vi "Periodic Tasks-Teleop Swerve.vi"(8 "error in":errorcluster) -> ()   [LabVIEW 2015]
doc: "This VI runs in parallel to other tasks. It can contain as many user-defined periodic loops as you need. These can carry out PID or other sorts of timed response."
uses:
  Robot Global Data.vi
  <vilib>/Rock Robotics/Network Tables/NT Read Number.vi
panel:
  out "Avg Absolute Distance":dbl
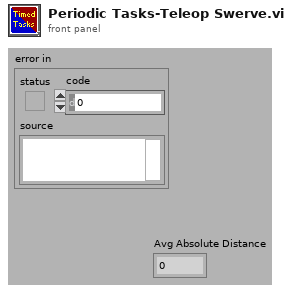
[diagram p1: front panel]
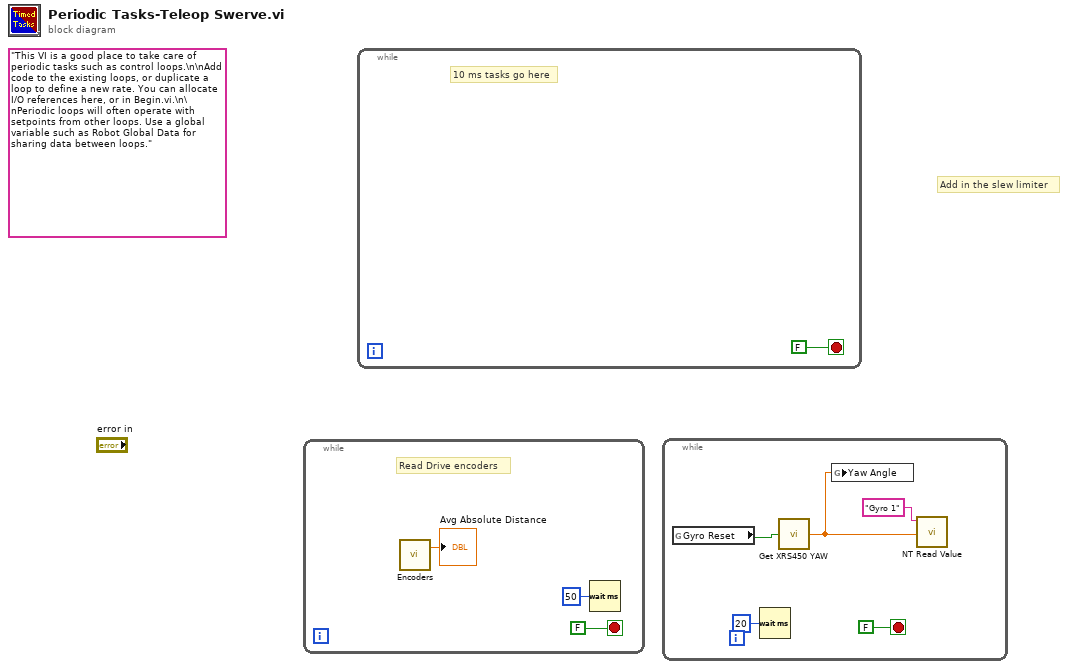
[diagram p0: block diagram]
diagram:
  (unwired) "This VI is a good place to take care of periodic tasks such as control loops.\n\nAdd code to the existing loops, or duplicate a loop to define a new rate. You can allocate I/O references here, or in Begin.vi.\n\nPeriodic loops will often operate with setpoints from other loops. Use a global variable such as Robot Global Data for sharing data between loops."
  # "Add in the slew limiter"
  n1 = while {
    stop <- FALSE stop-if-true
    # "Read Drive encoders"
    n2 = call "Encoders.vi"() -> ("Avg Absolute Distance"=→"Avg Absolute Distance":dbl)  [unwired: 2 in, 1 out]
    n3 = Wait (ms)(milliseconds to wait=u32 50) -> ()  [unwired: 1 out]
  }
  n4 = while {
    stop <- FALSE stop-if-true
    # "10 ms tasks go here"
  }
  n5 = while {
    stop <- FALSE stop-if-true
    n6 = global read "Robot Global Data.vi" "Gyro Reset"() -> (w8:bool)
    n7 = Wait (ms)(milliseconds to wait=u32 20) -> ()  [unwired: 1 out]
    n8 = call "Get XRS450 YAW.vi"("Reset Angle?"=w8) -> ("Angle"=w5:dbl)
    n9 = global write "Robot Global Data.vi" "Yaw Angle"(w5) -> ()
    n10 = call-poly <vilib>:"NT Read Value.vi"("Default Value"=w5, "Name"="Gyro 1") -> ()  [unwired: 8 in, 2 out]
  }
